vi "Run Resistivity of Bar sample Test.vi"(8 "error in (no error)":errorcluster) -> (0 "error out":errorcluster)   [LabVIEW 2016, in "Hall Effect Library.lvlib"]
uses:
  Hall Effect Library.lvlib
  Private/Test Procedures/Resistivity of Bar sample Test.vi
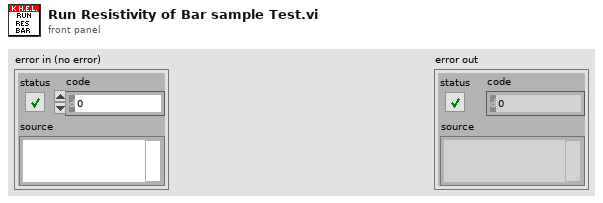
[diagram p1: front panel]
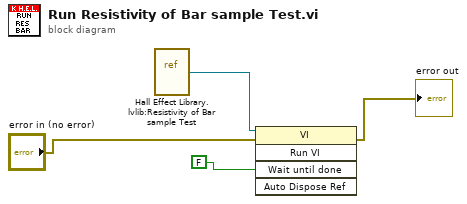
[diagram p0: block diagram]
diagram:
  n1 = vi-ref "Hall Effect Library.lvlib:Resistivity of Bar sample Test.vi"() -> (w4:refnum<vi>)
  n2 = invoke class="VI" method="Run VI"(reference=w4, error in="error in (no error)", "Wait until done"=FALSE) -> (error out=→"error out":errorcluster)  [unwired: 2 in, 4 out]
